vi "G#SubSubClass1_Create.vi"(0 "reference in":refnum<class "G#SubSubClass1.lvclass">, 2 "G#BaseClass1.lvclass":refnum<class "G#BaseClass1.lvclass">, 5 "error in (no error)":errorcluster) -> (14 "reference out":refnum<class "G#SubSubClass1.lvclass">, 19 "error out":errorcluster)   [LabVIEW 2017, in "G#SubSubClass1.lvclass"]
doc: "Constructor."
uses:
  G#SubSubClass1.lvclass
  C:/Program Files/National Instruments/LabVIEW 2017/vi.lib/addons/_AddQ/G#Object/G#Object.lvclass
  C:/Projects/GsharpGIT2017/Verification/TestCases/TestClasses/G#SubClass1_class/G#SubClass1.lvclass
  G#BaseClass1_class/G#BaseClass1.lvclass
  <vilib>/addons/_AddQ/G#Object/G#Object.lvclass
  G#SubClass1_class/G#SubClass1.lvclass
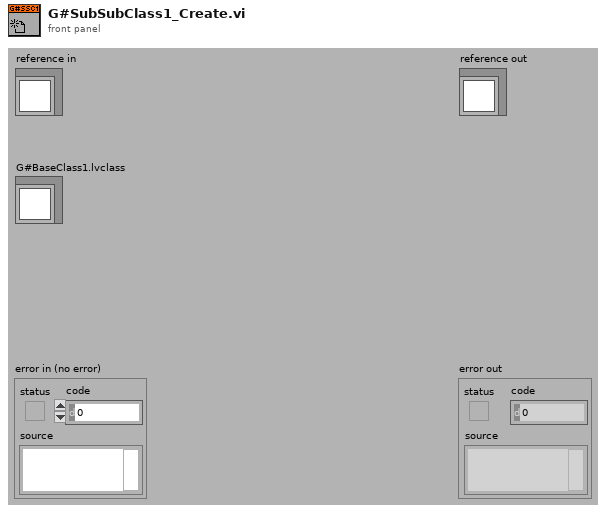
[diagram p1: front panel]
types:
  T1 = typedef "G#SubSubClass1.lvclass/ObjectAttributesRef.ctl" = refnum<data-value>
  T2 = typedef "G#SubSubClass1.lvclass/ObjectAttributes.ctl" = cluster{"Numeric":dbl, "G#BaseClass1.lvclass":refnum<class "G#BaseClass1.lvclass">}
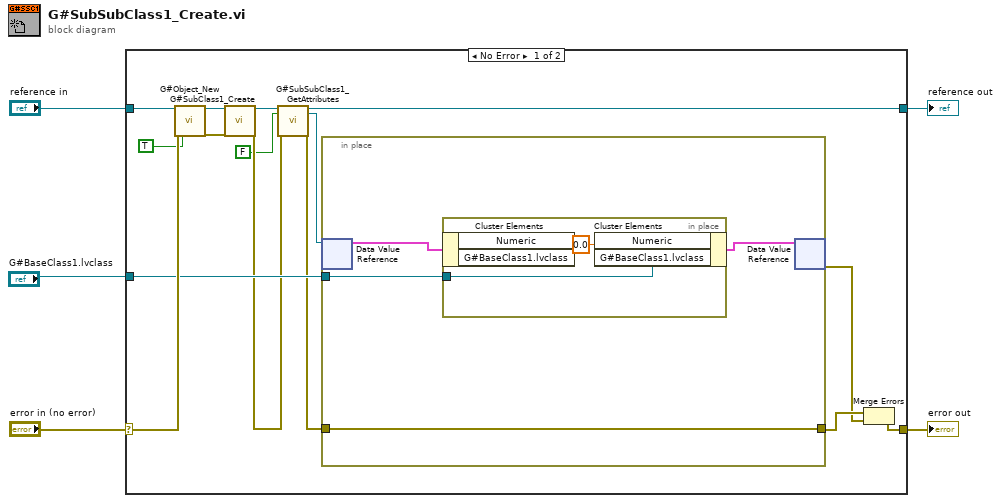
[diagram p0: block diagram]
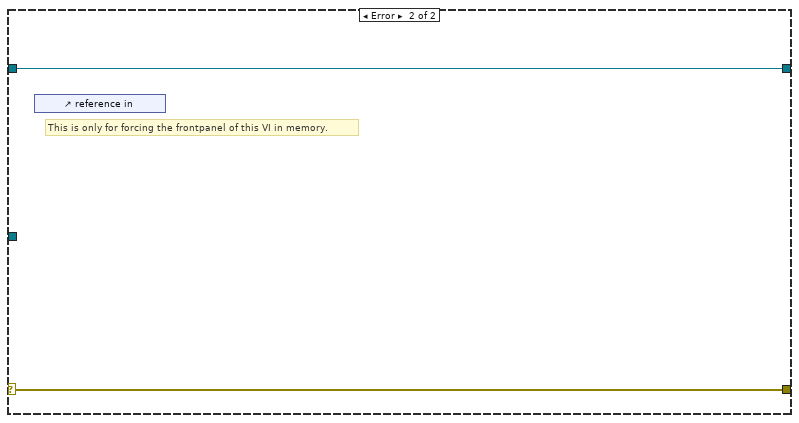
[diagram p2: hidden frame]
diagram:
  n1 = case shown="No Error" "error in (no error)" {
    selector: "error in (no error)" -> [w19 w28]
    tunnel: [w18 w28] -> w4
    tunnel: [w7 w27] -> w2
    tunnel: "reference in" -> [w20 w27]
    tunnel: "G#BaseClass1.lvclass" -> [w12 _]
    frame No Error {
      n2 = call <vilib>:"G#Object_New.vi"("reference in"=w20, "error in (no error)"=w19, "user counter (T)?"=TRUE ("User Counter")) -> ("reference out"=w17:refnum<class "G#SubSubClass1.lvclass">, "error out"=w16:errorcluster)  [unwired: 14 in, 1 out]
      n3 = call "G#SubClass1_Create.vi"("reference in"=w17, "error in (no error)"=w16) -> ("reference out"=w11:refnum<class "G#SubSubClass1.lvclass">, "error out"=w10:errorcluster)  [unwired: 15 in, 1 out]
      n4 = call "G#SubSubClass1_GetAttributes.vi"("reference in"=w11, "return data? (T)"=FALSE, "error in (no error)"=w10) -> ("reference out"=w7:refnum<class "G#SubSubClass1.lvclass">, "attributes ref"=w6:T1, "error out"=w9:errorcluster)  [unwired: 13 in, 1 out]
      n5 = in-place {
        in-place-border: w9 -> [w22]
        in-place-border: [w22] -> w14
        in-place-border: w12 -> [w21]
        n6 = in-place-dvr #1(w6) -> (w23:T2)  [unwired: 1 out]
        n7 = in-place {
          in-place-border: w21 -> [w25]
          n8 = in-place-cluster #2(w23) -> ()  [unwired: 2 out]
          n9 = in-place-cluster #2("Numeric"=0.0, "G#BaseClass1.lvclass"=w25) -> (w24:T2)
        }
        n10 = in-place-dvr #1(w24) -> (w13:errorcluster)  [unwired: 1 out]
      }
      n11 = Merge Errors(w14, w13) -> (w18:errorcluster)
    }
    frame Error {
      # "This is only for forcing the frontpanel of this VI in memory."
      n12 = control-ref of="reference in"() -> ()  [unwired: 1 out]
    }
  }
  "error out" <- w4
  "reference out" <- w2
